vi "SELECT COUNT SN.vi"(8 "errin":errorcluster, 10 "SN":string) -> (0 "error out":errorcluster, 3 "data":string)   [LabVIEW 2020]
doc: "Combien de fois le SN est'il present dans la base ?"
uses:
  <vilib>/addons/database/NI_Database_API.lvlib
  <vilib>/addons/database/Connection.llb/Conn Execute.vi
  <vilib>/addons/database/Recordset.llb/Rec Destroy - Connection.vi
  <vilib>/addons/database/Recordset.llb/Rec Fetch String Data (R).vi
  VarGLO/Global var.vi
  <vilib>/addons/database/Connection.llb/DB Tools Open Connec (String).vi
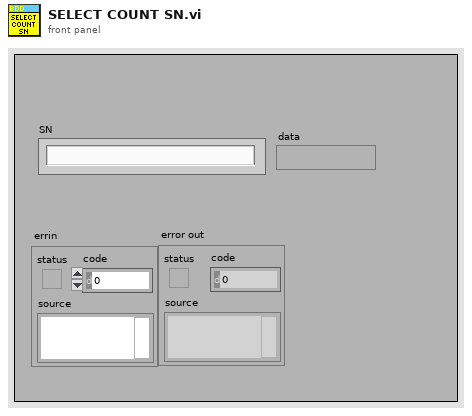
[diagram p1: front panel]
types:
  T1 = typedef "NI_Database_API.lvlib/Conn ObjectReference.ctl" = refnum<k1>
  T2 = typedef "NI_Database_API.lvlib/Rec ObjectReference.ctl" = refnum<k1>
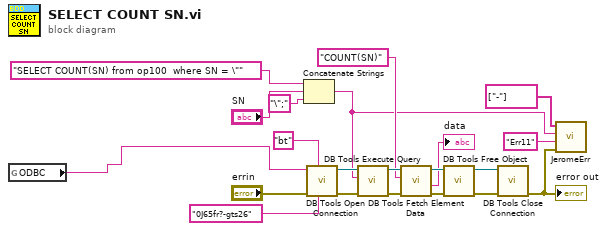
[diagram p0: block diagram]
diagram:
  n1 = global read "Global var.vi" "ODBC"() -> (w1:string)
  n2 = Concatenate Strings("SELECT COUNT(SN) from op100  where SN = \"" ("SQL query"), "SN", "\";" ("chaîne")) -> (w2:string)
  n3 = call-poly <vilib>:"DB Tools Open Connection.vi"("password"="0J65fr?-gts26", "userID"="bt", "error in (no error)"="errin", "connection information"=w1) -> ("error out"=w21:errorcluster, "connection reference"=w19:T1)  [unwired: 4 in]
  n4 = call-poly <vilib>:"DB Tools Execute Query.vi"("error in (no error)"=w21, "SQL query"=w2, "connection reference"=w19) -> ("error out"=w15:errorcluster, "recordset reference"=w14:T2)  [unwired: 5 in]
  n5 = call-poly <vilib>:"DB Tools Fetch Element Data.vi"("error in (no error)"=w15, "column index"="COUNT(SN)" ("type"), "recordset reference"=w14) -> ("error out"=w16:errorcluster, "data"=→"data":string, "recordset reference out"=w13:T2)  [unwired: 4 in]
  n6 = call-poly <vilib>:"DB Tools Free Object.vi"("error in (no error)"=w16, "recordset reference"=w13) -> ("error out"=w20:errorcluster, "connection reference"=w18:T1)  [unwired: 8 in]
  n7 = call <vilib>:"DB Tools Close Connection.vi"("error in (no error)"=w20, "connection reference"=w18) -> ("error out"=w3:errorcluster)  [unwired: 5 in]
  "error out" <- w3
  n8 = call "JeromeErr.vi"("Errin"=w3, "CodeERR"="Err11", "RequetteSQL"=w2, "RetourSQL"=string[] ["-"]) -> ()  [unwired: 8 in]
